vi "Save Back to the auto text file.vi"(9 "Path":path, 10 "Programs":string[](array[string]), 11 "Program Name":string[](array[string])) -> ()   [LabVIEW 2013]
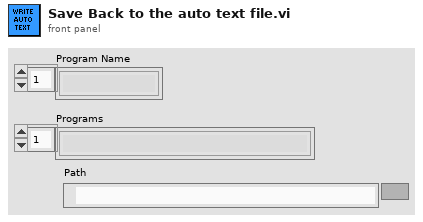
[diagram p1: front panel]
types:
  T1 = enum16{"open", "replace", "create", "open or create", "replace or create", "replace or create with confirmation"}
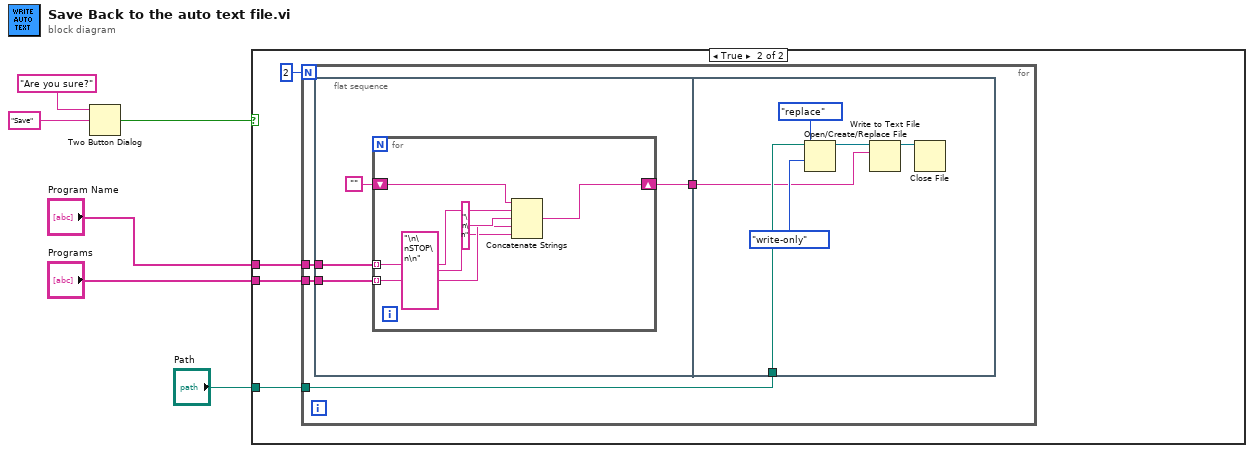
[diagram p0: block diagram]
diagram:
  n1 = Two Button Dialog(message="Are you sure?", 2:"Save" ("T button name (\"OK\")")) -> (T button?=w2:bool)  [unwired: 1 in]
  n2 = case shown="True" w2 {
    tunnel: "Programs" -> [_ w10]
    tunnel: "Program Name" -> [_ w9]
    tunnel: "Path" -> [_ w8]
    frame False {
    }
    frame True {
      n3 = for {
        N: 2 -> [_]
        tunnel: w10 -> [w13]
        tunnel: w9 -> [w12]
        tunnel: w8 -> [w11]
        n4 = flat-sequence {
          tunnel: w13 -> [w18]
          tunnel: w12 -> [w17]
          tunnel: [w15] -> w14
          tunnel: w11 -> [w29]
          tunnel: w14 -> [w26]
          frame #0 {
            n5 = for {
              tunnel: w17 -> [w23] mode=indexing
              tunnel: w18 -> [w21] mode=indexing
              shift-right: [w19] -> w15
              shift-left: "" -> [w24]
              n6 = Concatenate Strings(w24, w23, "\n\n" ("string"), w21, "\n\nSTOP\n\n" ("string")) -> (w19:string)
            }
          }
          frame #1 {
            n7 = Open/Create/Replace File(file path (use dialog)=w29, operation (0:open)=T1."replace", access (0:read/write)=enum16{"read/write", "read-only", "write-only"}."write-only") -> (refnum out=w28:refnum<file>)  [unwired: 3 in, 2 out]
            n8 = Write to Text File(file (use dialog)=w28, text=w26) -> (refnum out=w30:refnum<file>)  [unwired: 2 in, 2 out]
            n9 = Close File(refnum=w30) -> ()  [unwired: 1 in, 2 out]
          }
        }
      }
    }
  }
